vi "Configure Observer Logging.vi"(9 "Framework Instance Alias":string, 10 "Event Log Instance":refnum<class "LoggerReference.lvclass">, 11 "IObserver In":refnum<class "IObserver.lvclass">) -> (3 "IObserver Out":refnum<class "IObserver.lvclass">)   [LabVIEW 2017, in "IObserver.lvlib" / "IObserver.lvclass"]
doc: "<License>\nCopyright © 2017 Composed Systems, LLC | All rights reserved\nwww.composed.io\n\nAuthor: Ethan Stern <ethan.stern@composed.io>\n\nThis software is provided \"AS IS\" WITHOUT WARRANTIES, either express or implied, AND IS FOR EDUCATIONAL PURPOSES ONLY.\n</License>"
uses:
  IObserver.lvclass
  gpm_packages/@cs/event-logger/Source/Composed Log/LoggerReference/LoggerReference.lvclass
  IObserver.lvclass/IObserver.ctl
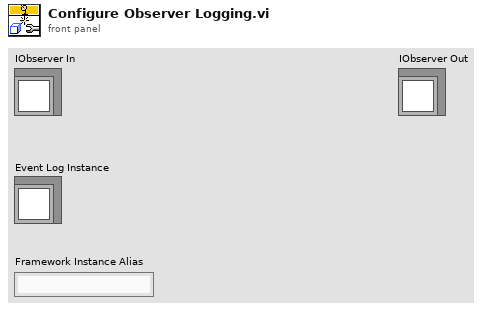
[diagram p1: front panel]
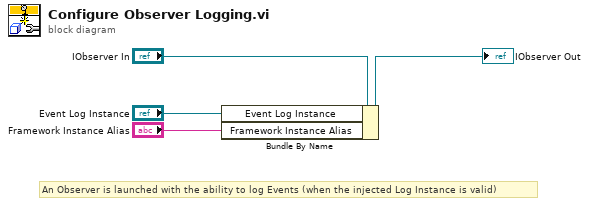
[diagram p0: block diagram]
diagram:
  # "An Observer is launched with the ability to log Events (when the injected Log Instance is valid)"
  n1 = Bundle By Name(cluster="IObserver In", "Event Log Instance"="Event Log Instance", "Framework Instance Alias"="Framework Instance Alias") -> (→"IObserver Out":refnum<class "IObserver.lvclass">)
